vi "Door Closed Interlock Value Change.vi"(8 "error in (no error)":errorcluster, 10 "Door Closed Interlock":bool, 11 "Doors Closed in":refnum<class "Doors Closed.lvclass">) -> (0 "error out":errorcluster, 3 "Doors Closed out":refnum<class "Doors Closed.lvclass">)   [LabVIEW 2020, in "Door Controller.lvlib" / "Doors Closed.lvclass"]
uses:
  Doors Closed.lvclass
  C:/Users/Thomas.McQuillan/Desktop/Elevator Door Control/Door Controller/Door Controller/Door Controller.lvclass
  Application/Application/Interlock Names.ctl
  Door Controller/Door Controller.lvclass
  Application/Application.lvlib
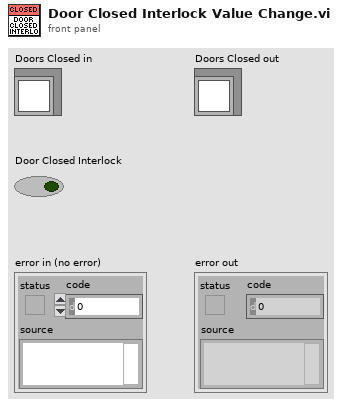
[diagram p1: front panel]
types:
  T1 = typedef "Application.lvlib/Interlock Names.ctl" = enum16{"Door Closed Interlock", "Door Open Interlock"}
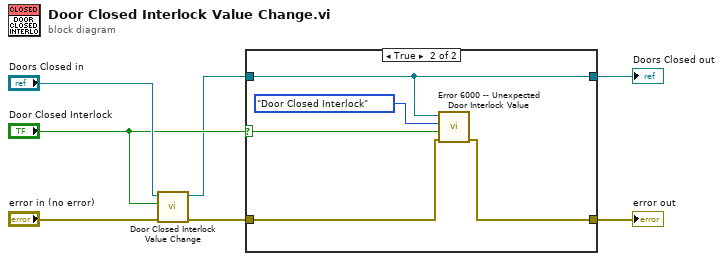
[diagram p0: block diagram]
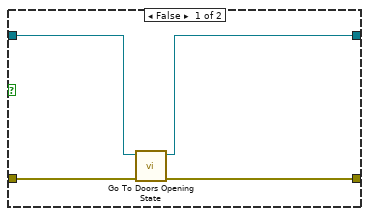
[diagram p2: hidden frame]
diagram:
  n1 = call-parent "Door Closed Interlock Value Change.vi"("error in (no error)"="error in (no error)", "Door Closed Interlock"="Door Closed Interlock", "Door Controller in"="Doors Closed in") -> ("error out"=w1:errorcluster, "Door Controller out"=w4:refnum<class "Doors Closed.lvclass">)  [unwired: 7 in]
  n2 = case shown="True" "Door Closed Interlock" {
    selector: "Door Closed Interlock" -> [_ w15]
    tunnel: w4 -> [w11 w16]
    tunnel: [w10 w16] -> w3
    tunnel: [w8 w12] -> w2
    tunnel: w1 -> [w9 w13]
    frame False {
      n3 = call "Go To Doors Opening State.vi"("error in (no error)"=w9, "Door Controller in"=w11) -> ("error out"=w8:errorcluster, "Door Controller out"=w10:refnum<class "Doors Closed.lvclass">)  [unwired: 8 in]
    }
    frame True {
      n4 = call "Error 6000 -- Unexpected Door Interlock Value.vi"("error in (no error)"=w13, "Interlock Value"=w15, "Interlock Name"=Interlock_Names."Door Closed Interlock", "Door Controller"=w16) -> ("error out"=w12:errorcluster)  [unwired: 7 in]
    }
  }
  "error out" <- w2
  "Doors Closed out" <- w3
